vi "Factorial of 5 number using structures with shift registers in LabVIEW.vi"() -> ()   [LabVIEW 2026]
panel:
  out "OUTPUT":dbl
  out "OUTPUT":dbl
  # "FOR loop"
  # "WHILE loop"
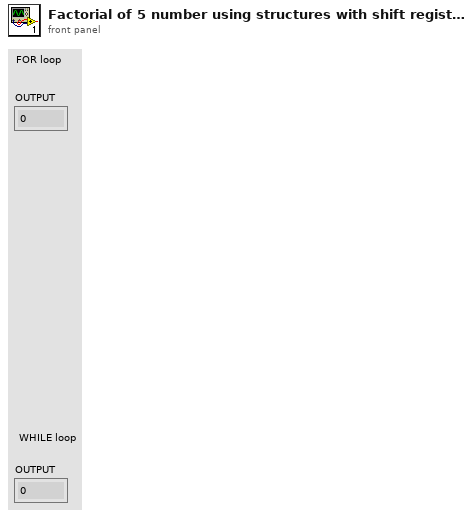
[diagram p1: front panel]
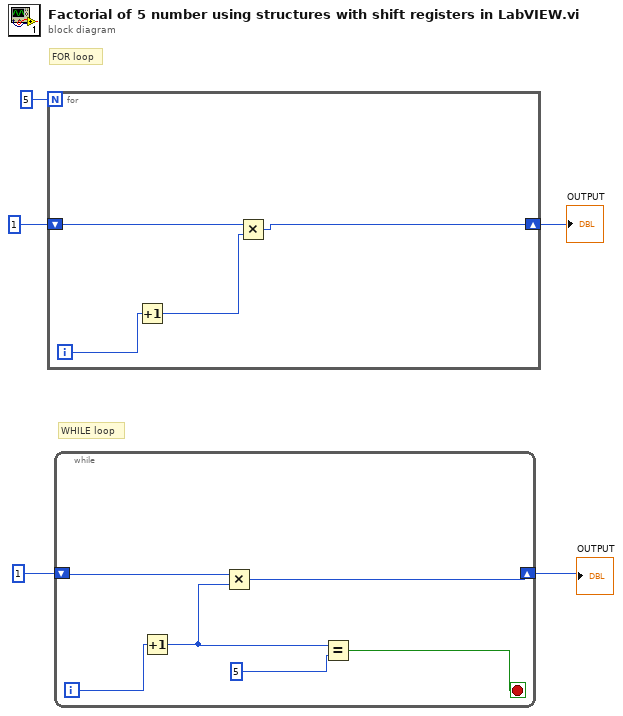
[diagram p0: block diagram]
diagram:
  # "WHILE loop"
  # "FOR loop"
  n1 = for {
    N: 5 -> [_]
    shift-right: [w6] -> w3
    shift-left: 1 -> [w9]
    i -> [w8]
    n2 = Increment(x=w8) -> (x+1=w7:i32)
    n3 = Multiply(x=w9, y=w7) -> (x*y=w6:i32)
  }
  "OUTPUT" <- w3
  n4 = while {
    shift-right: [w13] -> w1
    shift-left: 1 -> [w14]
    i -> [w15]
    stop <- w10 stop-if-true
    n5 = Increment(x=w15) -> (x+1=w12:i32)
    n6 = Multiply(x=w14, y=w12) -> (x*y=w13:i32)
    n7 = Equal?(x=w12, y=5) -> (x = y?=w10:bool)
  }
  "OUTPUT" <- w1
